vi "cDLTS temperature not stable.vi"(9 "Stabilization rate":dbl, 10 "Current sample temperature":dbl[unit], 11 "Temperature history in":T1) -> (2 "Temperature not stable":bool, 3 "Temperature history out":T1)   [LabVIEW 2019]
uses:
  <vilib>/Analysis/NI_AALPro.lvlib
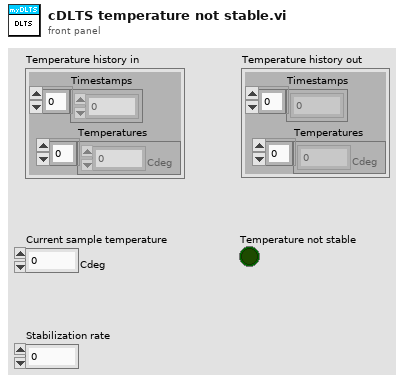
[diagram p1: front panel]
types:
  T1 = cluster{"Timestamps":ext[], "Temperatures":dbl[unit][]}
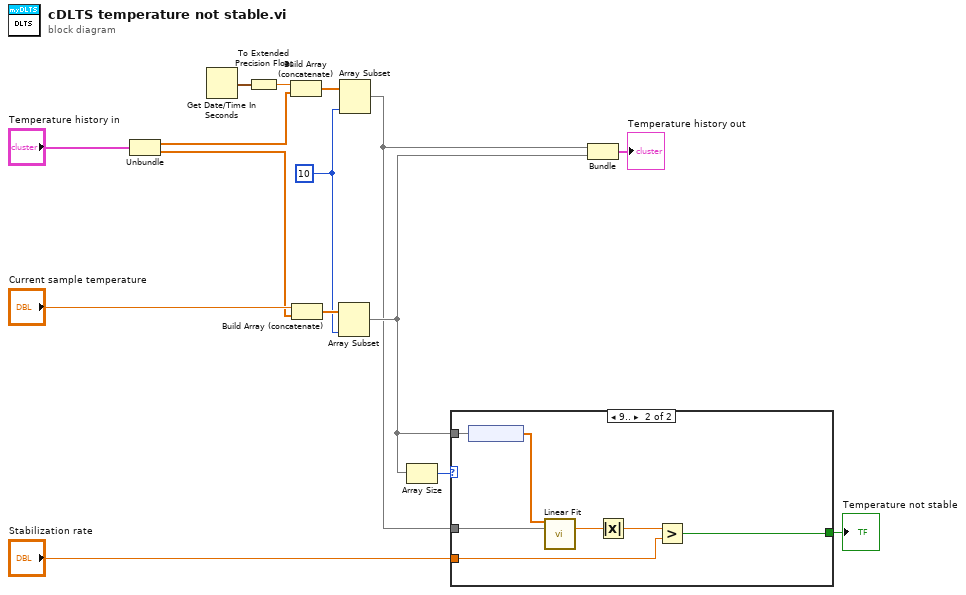
[diagram p0: block diagram]
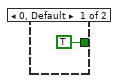
[diagram p2: hidden frame]
diagram:
  w12 = 10 ("length")
  n1 = Unbundle("Temperature history in") -> ("Timestamps"=w7:ext[], "Temperatures"=w6:dbl[unit][])
  n2 = Get Date/Time In Seconds() -> (seconds since 1Jan1904=w11:timestamp)
  n3 = To Extended Precision Float(1:w11) -> (0:w10:ext)
  n4 = Build Array (concatenate)(w10, w7) -> (w13:ext[])
  n5 = Build Array (concatenate)("Current sample temperature", w6) -> (w15:dbl[unit][])
  n6 = Array Subset(array=w15, length=w12) -> (w5:dbl[unit][])  [unwired: 1 in]
  n7 = Array Subset(array=w13, length=w12) -> (w3:ext[])  [unwired: 1 in]
  n8 = Array Size(array=w5) -> (size(s)=w4:i32)
  n9 = case shown="9.." w4 {
    tunnel: w5 -> [_ w23]
    tunnel: w3 -> [_ w21]
    tunnel: "Stabilization rate" -> [_ w18]
    tunnel: [TRUE w17] -> w1
    frame 0, Default {
    }
    frame 9.. {
      n10 = node(w23) -> (w22:dbl[])
      n11 = call <vilib>:"Linear Fit.vi"("Y"=w22, "X"=w21) -> ("slope"=w20:dbl)  [unwired: 9 in, 4 out]
      n12 = Absolute Value(x=w20) -> (abs(x)=w19:dbl)
      n13 = Greater?(x=w19, y=w18) -> (0:w17:bool)
    }
  }
  "Temperature not stable" <- w1
  n14 = Bundle(w3, w5) -> (→"Temperature history out":cluster{ext[], dbl[unit][]})  [unwired: 1 in]
